vi "ScaleY.vi"(9 "Time has Elapsed":bool, 10 "Length set point [mm]":dbl, 11 "WaveformChart in":refnum<vi>) -> (0 "error out":errorcluster)   [LabVIEW 2013]
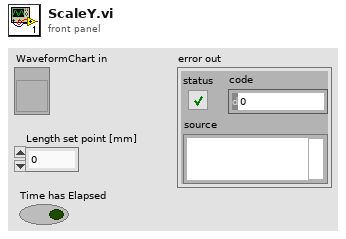
[diagram p1: front panel]
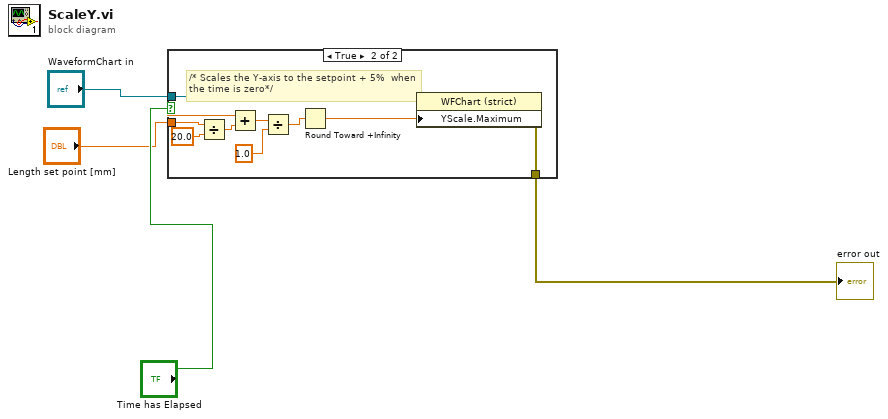
[diagram p0: block diagram]
diagram:
  n1 = case shown="True" "Time has Elapsed" {
    tunnel: [_ w13] -> w2
    tunnel: "Length set point [mm]" -> [_ w12]
    tunnel: "WaveformChart in" -> [_ w6]
    frame False {
    }
    frame True {
      # "/* Scales the Y-axis to the setpoint + 5%  when the time is zero*/"
      n2 = Divide(x=w12, y=20.0) -> (x/y=w10:dbl)
      n3 = Add(x=w12, y=w10) -> (x+y=w9:dbl)
      n4 = Divide(x=w9, y=1.0) -> (x/y=w8:dbl)
      n5 = Round Toward +Infinity(x=w8) -> (ceil(x): smallest int >= x=w5:dbl)
      n6 = property on="Property Node" class="WFChart (strict)"(reference=w6, "YScale.Maximum"=w5) -> (error out=w13:errorcluster)  [unwired: 1 in, 1 out]
    }
  }
  "error out" <- w2
